vi "DecodeRobotReplacement.vi"(1 "element":u8[](array[numeric]), 5 "error in (no error)":errorcluster) -> (15 "element 2":u8[](array[numeric]), 17 "repeated RobotReplacement":T1, 19 "error out":errorcluster)   [LabVIEW 2023, in "Referee.lvclass"]
uses:
  Referee.lvclass
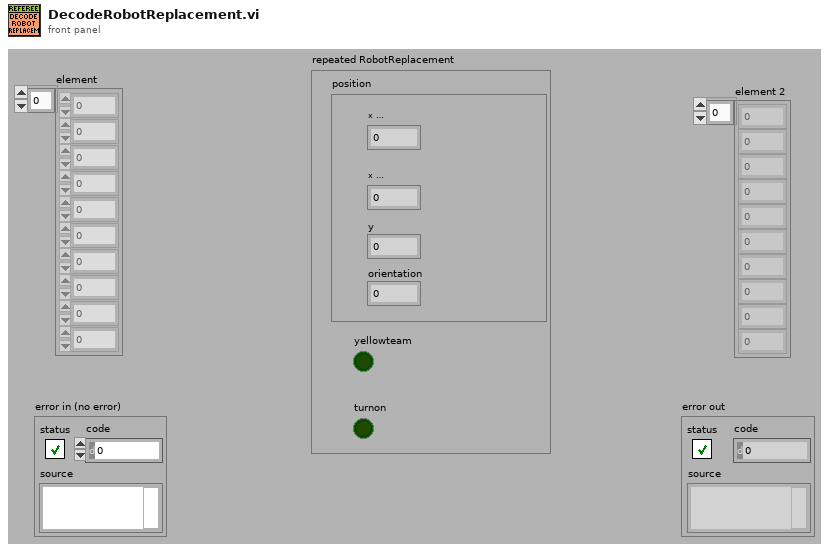
[diagram p1: front panel]
types:
  T1 = cluster{"position":cluster{"x\nx\nrobot_id":dbl, "x\nx\nx":dbl, "y":dbl, "orientation":dbl}, "yellowteam":bool, "turnon":bool}
  T2 = cluster{"robot_id":dbl, "x":dbl, "y":dbl, "orientation":dbl}
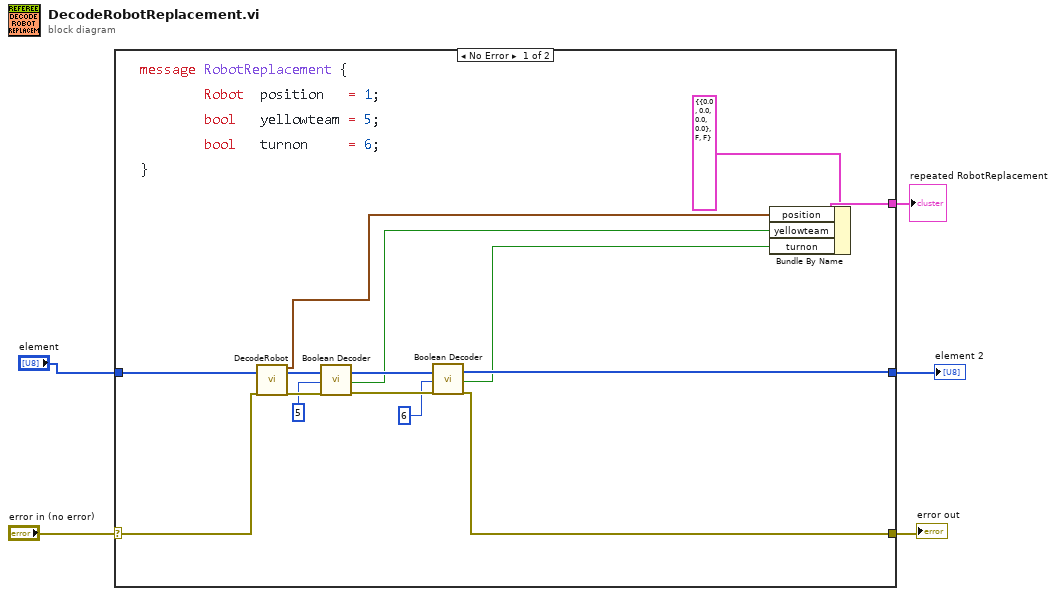
[diagram p0: block diagram]
diagram:
  n1 = case shown="No Error" "error in (no error)" {
    selector: "error in (no error)" -> [w19 w21]
    tunnel: [w12 w21] -> w4
    tunnel: [w11 _] -> w3
    tunnel: "element" -> [w20 _]
    tunnel: [w10 _] -> w1
    frame No Error {
      n2 = call "DecodeRobot.vi"("element"=w20, "error in (no error)"=w19) -> ("position"=w6:T2, "element 2"=w15:u8[], "error out"=w18:errorcluster)  [unwired: 15 in]
      n3 = call "Boolean Decoder.vi"("array"=w15, "Key"=5, "error in (no error)"=w18) -> ("array w/ subset deleted"=w13:u8[], "Bool"=w7:bool, "error out"=w17:errorcluster)  [unwired: 14 in]
      n4 = call "Boolean Decoder.vi"("array"=w13, "Key"=6, "error in (no error)"=w17) -> ("array w/ subset deleted"=w11:u8[], "Bool"=w8:bool, "error out"=w12:errorcluster)  [unwired: 14 in]
      n5 = Bundle By Name(cluster=T1 {"position"={"x\nx\nrobot_id"=0.0, "x\nx\nx"=0.0, "y"=0.0, "orientation"=0.0}, "yellowteam"=FALSE, "turnon"=FALSE} ("repeated RobotReplacement 2"), "position"=w6, "yellowteam"=w7, "turnon"=w8) -> (w10:T1)
    }
    frame Error {
    }
  }
  "error out" <- w4
  "element 2" <- w3
  "repeated RobotReplacement" <- w1
